vi "PMX_HoldPeakValues.vi"(0 "Device":refnum<k24>, 1 "Signal":refnum<k24>, 2 "HoldMin":bool=TRUE, 3 "HoldMax":bool=TRUE, 4 "HoldPeakToPeak":bool=TRUE, 5 "Error in":errorcluster) -> (14 "Device":refnum<k24>, 19 "Error out":errorcluster)   [LabVIEW 2016]
doc: "Holds or enables peak value function (min, max, peak to peak) of the given signal.\n\nSignal: Signal for which peak should be enabled/disabled \nHoldMin: Set to true, if minimum value should be frozen (default value is true)\nHoldMax: Set to true, if maximum value should be frozen (default value is true)\nHoldPeakToPeak: Set to true, if peak to peak value should be frozen (default value is true)"
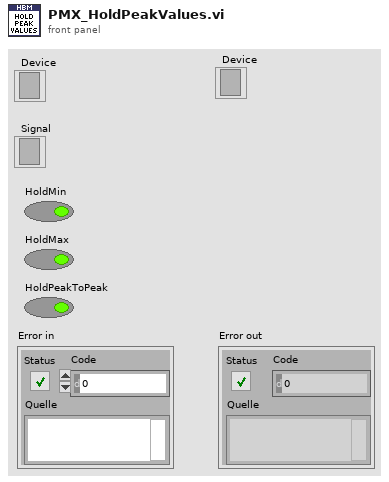
[diagram p1: front panel]
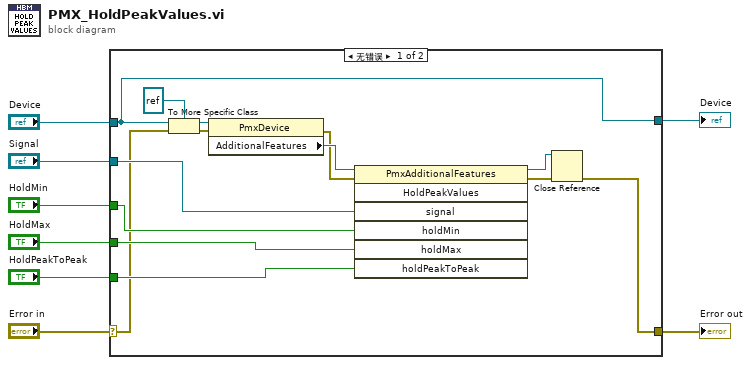
[diagram p0: block diagram]
diagram:
  n1 = case shown="无错误" "Error in" {
    selector: "Error in" -> [w13 w24]
    tunnel: [w10 w24] -> w6
    tunnel: "Device" -> [w18 w23]
    tunnel: [w18 w23] -> w7
    tunnel: "Signal" -> [w17 _]
    tunnel: "HoldPeakToPeak" -> [w16 _]
    tunnel: "HoldMax" -> [w15 _]
    tunnel: "HoldMin" -> [w14 _]
    frame No Error {
      n2 = To More Specific Class(target class=refnum<k24> refnum ("Zielklasse"), reference=w18, error in=w13) -> (specific class reference=w22:refnum<k24>, error out=w19:errorcluster)
      n3 = property on="Eigenschaftsknoten" class="PmxDevice"(reference=w22, error in=w19) -> (error out=w20:errorcluster, "AdditionalFeatures"=w21:refnum<k24>)  [unwired: 1 out]
      n4 = invoke on="Methodenknoten" class="PmxAdditionalFeatures" method="HoldPeakValues"(reference=w21, error in=w20, "signal"=w17, "holdMin"=w14, "holdMax"=w15, "holdPeakToPeak"=w16) -> (reference out=w9:refnum<k24>, error out=w11:errorcluster)  [unwired: 1 in, 5 out]
      n5 = Close Reference(reference=w9, error in (no error)=w11) -> (error out=w10:errorcluster)
    }
    frame Error {
    }
  }
  "Device" <- w7
  "Error out" <- w6
